vi "add string to path.vi"(9 "String":string, 11 "path":path) -> (3 "appended path":path)   [LabVIEW 2014]
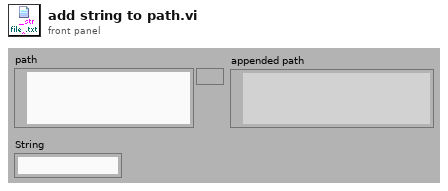
[diagram p1: front panel]
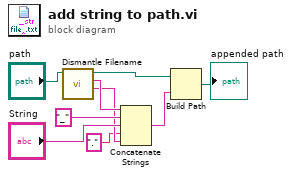
[diagram p0: block diagram]
diagram:
  n1 = call "Dismantle Filename.vi"("file"="path") -> ("lowercase file extension"=w2:string, "file name without extension"=w7:string, "stripped path"=w8:path)  [unwired: 3 in, 1 out]
  n2 = Concatenate Strings(w7, "_" ("string"), "String", "." ("string"), w2) -> (w6:string)
  n3 = Build Path(base path=w8, name or relative path=w6) -> (appended path=→"appended path":path)
